vi "Lower_Stop.vi"(8 "error in (no error)":errorcluster, 10 "I-O in":refnum<class "I-O.lvclass">, 11 "Motion in":refnum<class "Motion.lvclass">) -> (0 "error out":errorcluster, 2 "I-O out":refnum<class "I-O.lvclass">, 3 "Motion out":refnum<class "Motion.lvclass">)   [LabVIEW 2016]
uses:
  Classes/Controller/Motion/Motion Folder/Motion.lvclass
  Classes/Controller/I-O/I-O Folder/I-O.lvclass
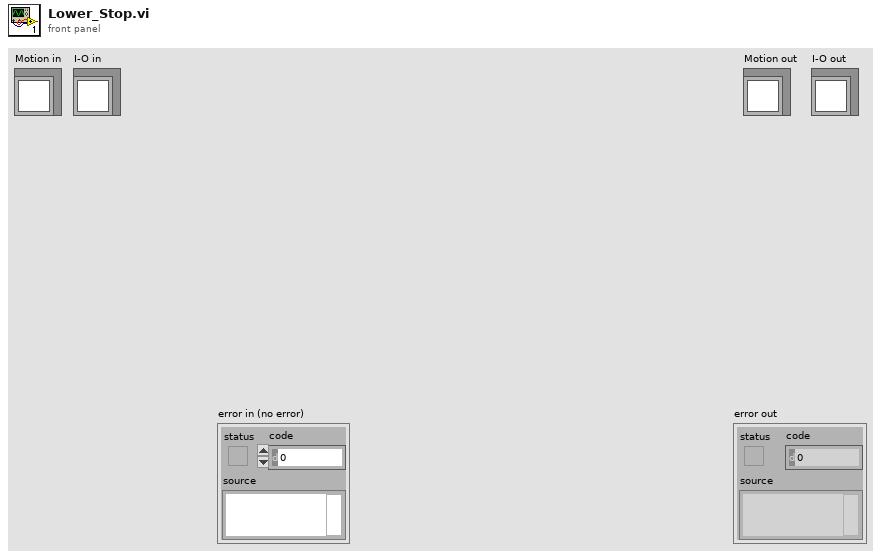
[diagram p1: front panel]
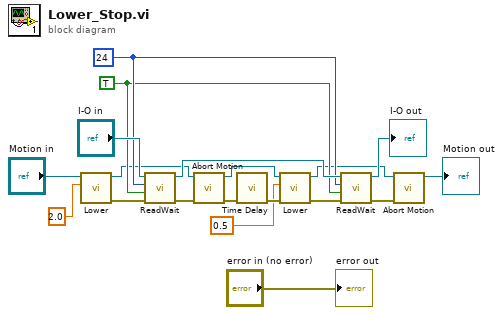
[diagram p0: block diagram]
diagram:
  w12 = TRUE ("Value")
  w13 = 24 ("Read")
  n1 = call-dynamic "Lower.vi"("Speed"=2.0, "Motion in"="Motion in") -> ("error out"=w19:errorcluster, "Motion out"=w5:refnum<class "Motion.lvclass">)  [unwired: 8 in]
  n2 = call "ReadWait.vi"("error in (no error)"=w19, "Value"=w12, "Read"=w13, "I-O in"="I-O in") -> ("error out"=w6:errorcluster, "I-O out"=w14:refnum<class "I-O.lvclass">)  [unwired: 6 in]
  n3 = call-dynamic "Abort Motion.vi"("error in (no error)"=w6, "Motion in"=w5) -> ("error out"=w4:errorcluster, "Motion out"=w2:refnum<class "Motion.lvclass">)  [unwired: 8 in]
  n4 = call "Time Delay"("error in (no error)"=w4) -> ("error out"=w3:errorcluster)  [unwired: 10 in]
  n5 = call-dynamic "Lower.vi"("error in (no error)"=w3, "Speed"=0.5, "Motion in"=w2) -> ("error out"=w9:errorcluster, "Motion out"=w7:refnum<class "Motion.lvclass">)  [unwired: 7 in]
  n6 = call "ReadWait.vi"("error in (no error)"=w9, "Value"=w12, "Read"=w13, "I-O in"=w14) -> ("error out"=w10:errorcluster, "I-O out"=→"I-O out":refnum<class "I-O.lvclass">)  [unwired: 6 in]
  n7 = call-dynamic "Abort Motion.vi"("error in (no error)"=w10, "Motion in"=w7) -> ("Motion out"=→"Motion out":refnum<class "Motion.lvclass">)  [unwired: 8 in, 1 out]
  "error out" <- "error in (no error)"
